vi "Word_LVtoWD_Color.vi"(1 "LabVIEW color":u32(colorbox)) -> (0 "word color table index":i32)   [LabVIEW 2010, in "NI_ReportGenerationToolkit.lvlib"]
uses:
  <vilib>/addons/_office/NI_ReportGenerationToolkit.lvlib
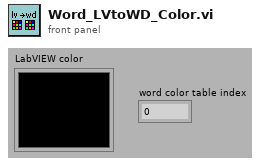
[diagram p1: front panel]
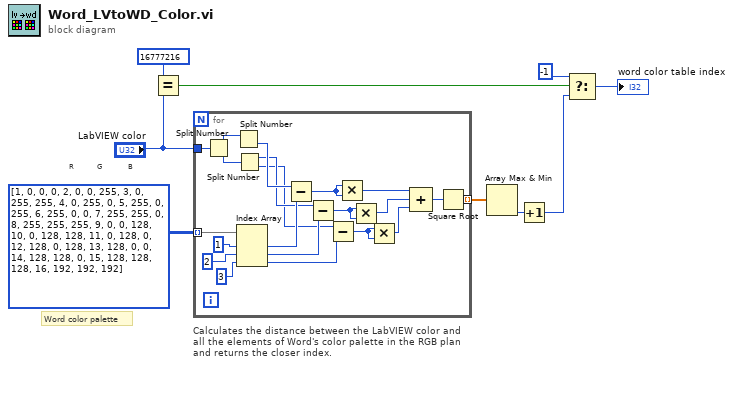
[diagram p0: block diagram]
diagram:
  # "Calculates the distance between the LabVIEW color and all the elements of Word's color palette in the RGB plan and returns the closer index."
  # "B"
  # "G"
  # "R"
  # "Word color palette"
  n1 = Equal?(x=16777216, y="LabVIEW color") -> (x = y?=w5:bool)
  n2 = for {
    tunnel: i32[][] [[1, 0, 0, 0], [2, 0, 0, 255], [3, 0, 255, 255], [4, 0, 255, 0], [5, 255, 0, 255], [6, 255, 0, 0], [7, 255, 255, 0], [8, 255, 255, 255], [9, 0, 0, 128], [10, 0, 128, 128], [11, 0, 128, 0], [12, 128, 0, 128], [13, 128, 0, 0], [14, 128, 128, 0], [15, 128, 128, 128], [16, 192, 192, 192]] ("data") -> [w28] mode=indexing
    tunnel: [w10] -> w9 mode=indexing
    tunnel: "LabVIEW color" -> [w17]
    n3 = Split Number(x=w17) -> (hi(x)=w30:u16, lo(x)=w29:u16)
    n4 = Split Number(x=w30) -> (lo(x)=w21:u8)  [unwired: 1 out]
    n5 = Split Number(x=w29) -> (hi(x)=w20:u8, lo(x)=w19:u8)
    n6 = Index Array(array=w28, index #1=1 ("Index"), index #2=2 ("Index"), index #3=3 ("Index")) -> (element #1=w22:i32, element #2=w23:i32, element #3=w24:i32)
    n7 = Subtract(x=w21, y=w22) -> (x-y=w16:i32)
    n8 = Subtract(x=w20, y=w23) -> (x-y=w14:i32)
    n9 = Subtract(x=w19, y=w24) -> (x-y=w15:i32)
    n10 = Multiply(x=w16, y=w16) -> (x*y=w13:i32)
    n11 = Multiply(x=w14, y=w14) -> (x*y=w12:i32)
    n12 = Multiply(x=w15, y=w15) -> (x*y=w11:i32)
    n13 = Compound Arithmetic op=ADD(w13, w12, w11) -> (w18:i32)
    n14 = Square Root(x=w18) -> (sqrt(x)=w10:dbl)
  }
  n15 = Array Max & Min(array=w9) -> (min index (indices)=w8:i32)  [unwired: 3 out]
  n16 = Increment(x=w8) -> (x+1=w1:i32)
  n17 = Select(t=-1, s=w5, f=w1) -> (s? t:f=→"word color table index":i32)
